vi "Send Method.vi"(7 "Message Priority (Normal)":enum16{"Low", "Normal", "High"}(ring)=enum."Normal", 8 "error in":errorcluster, 9 "String":string, 10 "Numeric":dbl, 11 "Message Enqueuer":refnum<class "Message Enqueuer.lvclass">) -> (0 "error out":errorcluster, 3 "Message Enqueuer out":refnum<class "Message Enqueuer.lvclass">)   [LabVIEW 2015, in "Main.lvlib" / "Method Msg.lvclass"]
doc: "This VI sends the message to an actor."
uses:
  Method Msg.lvclass
  <vilib>/ActorFramework/Message Enqueuer/Message Enqueuer.lvclass
  Method Msg.lvclass/Method Msg.ctl
  <vilib>/ActorFramework/Message Enqueuer/Message Enqueuer.lvclass/Message Enqueuer.ctl
  <vilib>/ActorFramework/Message Priority Queue/Priority Enqueue.vi
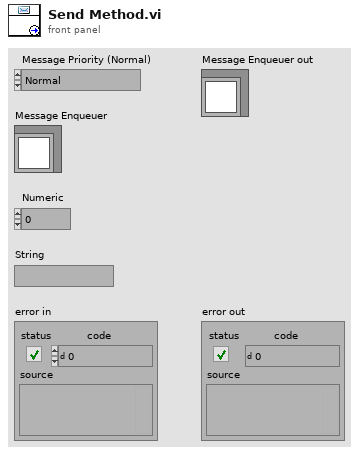
[diagram p1: front panel]
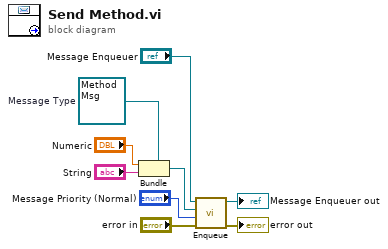
[diagram p0: block diagram]
diagram:
  w6 = refnum<class "Method Msg.lvclass"> refnum  # Message Type
  n1 = Bundle(cluster=w6, "Numeric", "String") -> (w5:refnum<class "Method Msg.lvclass">)
  n2 = call <vilib>:"Enqueue.vi"("error in"="error in", "Message Priority"="Message Priority (Normal)", "Message"=w5, "Message Enqueuer in"="Message Enqueuer") -> ("error out"=→"error out":errorcluster, "Message Enqueuer out"=→"Message Enqueuer out":refnum<class "Message Enqueuer.lvclass">)  [unwired: 6 in]
